vi "CFTS-Write Options.vi"(8 "error in (no error)":errorcluster, 11 "CFTS Options":T1) -> (0 "error out":errorcluster)   [LabVIEW 2020]
uses:
  CFTS-Options.ctl
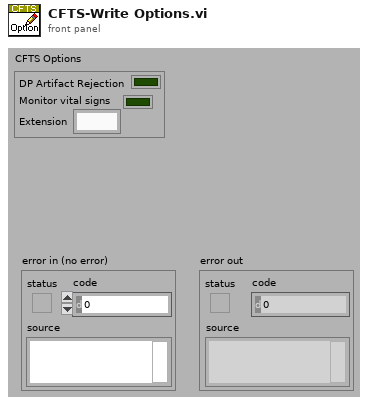
[diagram p1: front panel]
types:
  T1 = typedef "CFTS-Options.ctl" = cluster{"DP Artifact Rejection":bool, "Monitor vital signs ":bool, "Extension":string}
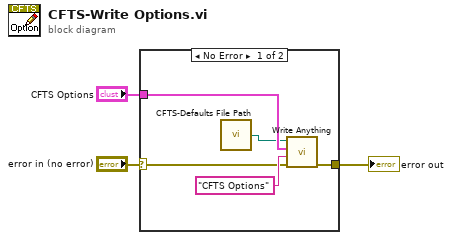
[diagram p0: block diagram]
diagram:
  n1 = case shown="No Error" "error in (no error)" {
    selector: "error in (no error)" -> [w7 w9]
    tunnel: [w5 w9] -> w3
    tunnel: "CFTS Options" -> [w6 _]
    frame No Error {
      n2 = call "CFTS-Defaults File Path.vi"() -> ("Path"=w4:path)  [unwired: 1 in]
      n3 = call "Write Anything.vi"("Error In"=w7, "Section Name (Name of \"Anything\")"="CFTS Options" ("Section Name (Name of \"Type of Anything\")"), "Anything"=w6, "Path (dialog)"=w4) -> ("Error Out"=w5:errorcluster)  [unwired: 6 in, 1 out]
    }
    frame Error {
    }
  }
  "error out" <- w3
